vi "RestartSafety.vi"(0 "Universal Robot.lvclass in":refnum<class "Universal Robot.lvclass">, 5 "error in (no error)":errorcluster) -> (14 "Universal Robot.lvclass out":refnum<class "Universal Robot.lvclass">, 19 "error out":errorcluster)   [LabVIEW 2016, in "Universal Robot.lvclass"]
uses:
  Universal Robot.lvclass
  Universal Robot.lvclass/Universal Robot.ctl
  SafetyStatus.ctl
  DashboardServer/Dashboard Server.lvclass
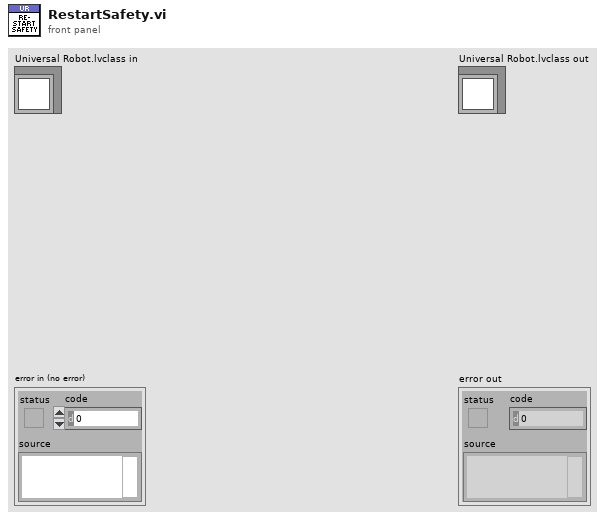
[diagram p1: front panel]
types:
  T1 = typedef "Universal Robot.lvclass/SafetyStatus.ctl" = enum16{"INVALID", "NORMAL", "REDUCED", "PROTECTIVE_STOP", "RECOVERY", "SAFEGAURD_STOP", "SYSTEM_EMERGENCY_STOP", "ROBOT_EMERGENCY_STOP", "VIOLATION", "FAULT", "AUTOMATIC_MODE_SAFEGAURD_STOP", "SYSTEM_THREE_POSITION_ENABLING_STOP"}
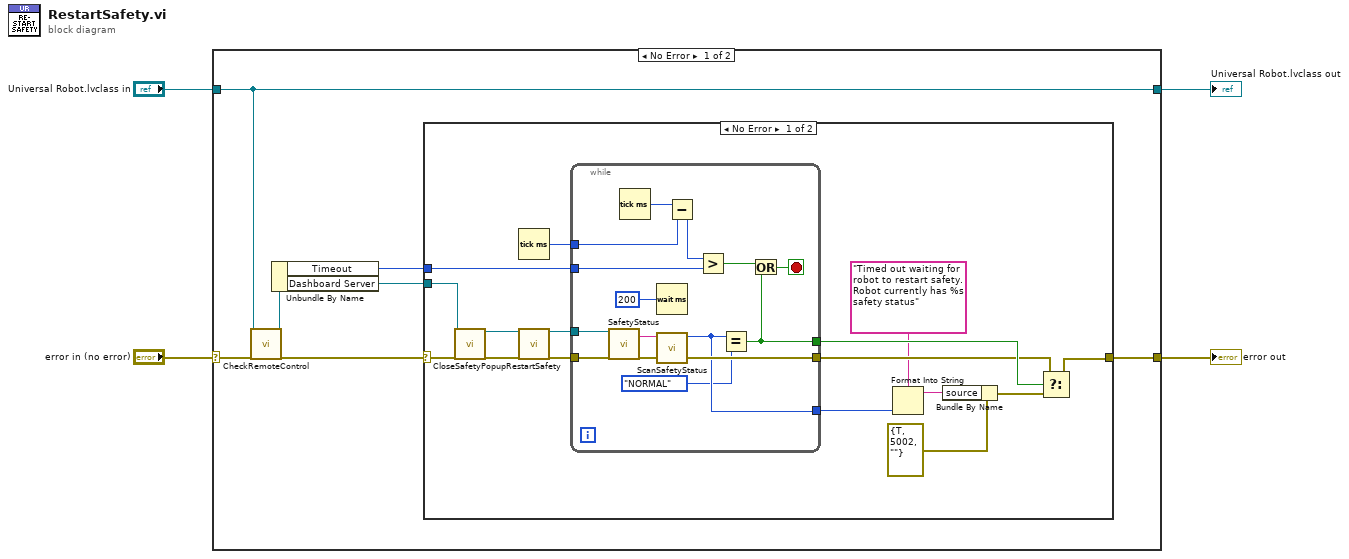
[diagram p0: block diagram]
diagram:
  n1 = case shown="No Error" "error in (no error)" {
    selector: "error in (no error)" -> [w10 w44]
    tunnel: [w11 w44] -> w3
    tunnel: "Universal Robot.lvclass in" -> [w9 w43]
    tunnel: [w9 w43] -> w1
    frame No Error {
      n2 = call-dynamic "CheckRemoteControl.vi"("Universal Robot.lvclass in"=w9, "error in (no error)"=w10) -> ("Universal Robot.lvclass out"=w8:refnum<class "Universal Robot.lvclass">, "error out"=w5:errorcluster)  [unwired: 16 in]
      n3 = Unbundle By Name(w8) -> ("Timeout"=w6:u32, "Dashboard Server"=w7:refnum<class "Dashboard Server.lvclass">)
      n4 = case shown="No Error" w5 {
        selector: w5 -> [w17 w42]
        tunnel: [w27 w42] -> w11
        tunnel: w7 -> [w16 _]
        tunnel: w6 -> [w26 _]
        frame No Error {
          n5 = call-dynamic "CloseSafetyPopup.vi"("DashboardServer in"=w16, "error in (no error)"=w17) -> ("DashboardServer out"=w15:refnum<class "Dashboard Server.lvclass">, "error out"=w14:errorcluster)  [unwired: 15 in, 1 out]
          n6 = Tick Count (ms)() -> (millisecond timer value=w25:u32)
          n7 = call-dynamic "RestartSafety.vi"("DashboardServer in"=w15, "error in (no error)"=w14) -> ("DashboardServer out"=w13:refnum<class "Dashboard Server.lvclass">, "error out"=w12:errorcluster)  [unwired: 15 in, 1 out]
          n8 = while {
            tunnel: [w33] -> w23
            tunnel: w26 -> [w40]
            tunnel: w25 -> [w39]
            tunnel: [w34] -> w24
            tunnel: [w29] -> w22
            tunnel: w13 -> [w32]
            tunnel: w12 -> [w31]
            stop <- w35 stop-if-true
            n9 = call-dynamic "SafetyStatus.vi"("DashboardServer in"=w32, "error in (no error)"=w31) -> ("safetyStatus"=w30:string, "error out"=w33:errorcluster)  [unwired: 15 in, 1 out]
            n10 = Tick Count (ms)() -> (millisecond timer value=w38:u32)
            n11 = Wait (ms)(milliseconds to wait=u32 200) -> ()  [unwired: 1 out]
            n12 = call "ScanSafetyStatus.vi"("safetyStatus in"=w30) -> ("safetyStatus out"=w29:T1)  [unwired: 10 in]
            n13 = Subtract(x=w38, y=w39) -> (x-y=w37:u32)
            n14 = Greater?(x=w37, y=w40) -> (0:w36:bool)
            n15 = Equal?(x=w29, y=SafetyStatus."NORMAL") -> (x = y?=w34:bool)
            n16 = Or(x=w36, y=w34) -> (x .or. y?=w35:bool)
          }
          n17 = Format Into String(format string="Timed out waiting for robot to restart safety. Robot currently has %s safety status", w22) -> (resulting string=w20:string)  [unwired: 2 in, 1 out]
          n18 = Bundle By Name(cluster=errorcluster {"status"=TRUE, "code"=5002, "source"=""} ("error constant"), "source"=w20) -> (w19:errorcluster)
          n19 = Select(t=w23, s=w24, f=w19) -> (s? t:f=w27:errorcluster)
        }
        frame Error {
        }
      }
    }
    frame Error {
    }
  }
  "error out" <- w3
  "Universal Robot.lvclass out" <- w1
